vi "VI Konfiguration Kalibriergase.vi"() -> ()   [LabVIEW 2020, in "CalGas Aufschaltung.lvlib"]
uses:
  Seiten/CalGas Aufschaltung/CalGas Aufschaltung.lvlib
  Seiten/CalGas Aufschaltung/Definition CalGas Anzeige.ctl
  Seiten/CalGas Aufschaltung/CalGas-Namen.ctl
  Visualisierungs Elemente/String - Eingabefeld.ctl
  Seiten/CalGas Aufschaltung/CalGas-Werte.ctl
  Visualisierungs Elemente/Zahlen-Eingabefeld.ctl
  Seiten/CalGas Aufschaltung/CalGas-Einheit.ctl
  Visualisierungs Elemente/Auswahlfeld.ctl
  Seiten/CalGas Aufschaltung/CalGas-Messbereiche.ctl
  Seiten/CalGas Aufschaltung/Aufschaltung CalGas_ANZEIGE.ctl
  Seiten/CalGas Aufschaltung/Cluster Auswahl Analysator.ctl
  Seiten/CalGas Aufschaltung/Analysator Auswahl.ctl
  Seiten/CalGas Aufschaltung/FGV CalGas Aktionen.ctl
  Passwortverwaltung/FGV Passwort Aktion.ctl
  Analysator Definition/FGV Analysator Definition Aktionen.ctl
  Passwortverwaltung/Passwort.lvlib
  Allgemein/allgemeine Sub-VIs.lvlib
  Analysator Definition/Analysator Definition.lvlib
panel:
  in  "Analysator Auswahl":T1 {"Analysator Auswahl 12" items=["----"=100, "FT-IR"=0, "TEST"=1]; "Analysator Auswahl 11" items=["----"=100, "FT-IR"=0, "TEST"=1]; "Analysator Auswahl 10" items=["----"=100, "FT-IR"=0, "TEST"=1]; "Analysator Auswahl 9" items=["----"=100, "FT-IR"=0, "TEST"=1]; "Analysator Auswahl 8" items=["----"=100, "FT-IR"=0, "TEST"=1]; "Analysator Auswahl 7" items=["----"=100, "FT-IR"=0, "TEST"=1]; "Analysator Auswahl 6" items=["----"=100, "FT-IR"=0, "TEST"=1]; "Analysator Auswahl 5" items=["----"=100, "FT-IR"=0, "TEST"=1]; "Analysator Auswahl 4" items=["----"=100, "FT-IR"=0, "TEST"=1]; "Analysator Auswahl 3" items=["----"=100, "FT-IR"=0, "TEST"=1]; "Analysator Auswahl 2" items=["----"=100, "FT-IR"=0, "TEST"=1]; "Analysator Auswahl" items=["----"=100, "FT-IR"=0, "PMA"=1]}
  in  "Aufschaltung CalGas":T3 {"Aufschaltpunkt" items=["Filterblock", "Analyzer directly", "PNS", "Entnahme", "Gasdivider"]; "Kalibriergas" items=["Stickstoff"]}
  in  "Def.CalGas":T5 {"Messbereiche"."Messbereich 12" items=["---"]; "Messbereiche"."Messbereich 11" items=["---"]; "Messbereiche"."Messbereich 10" items=["---"]; "Messbereiche"."Messbereich 9" items=["---"]; "Messbereiche"."Messbereich 8" items=["---"]; "Messbereiche"."Messbereich 7" items=["---"]; "Messbereiche"."Messbereich 6" items=["---"]; "Messbereiche"."Messbereich 5" items=["---"]; "Messbereiche"."Messbereich 4" items=["---"]; "Messbereiche"."Messbereich 3" items=["---"]; "Messbereiche"."Messbereich 2" items=["---"]; "Messbereiche"."Messbereich 1" items=["---"]; "Einheit"."Einheit 12" items=["ppm", "%"]; "Einheit"."Einheit 11" items=["ppm", "%"]; "Einheit"."Einheit 10" items=["ppm", "%"]; "Einheit"."Einheit 9" items=["ppm", "%"]; "Einheit"."Einheit 8" items=["ppm", "%"]; "Einheit"."Einheit 7" items=["ppm", "%"]; "Einheit"."Einheit 6" items=["ppm", "%"]; "Einheit"."Einheit 5" items=["ppm", "%"]; "Einheit"."Einheit 4" items=["ppm", "%"]; "Einheit"."Einheit 3" items=["ppm", "%"]; "Einheit"."Einheit 2" items=["ppm", "%"]; "Einheit"."Einheit 1" items=["ppm", "%"]; "Werte 2"."Konzentration 12" format="%#_5g"; "Werte 2"."Konzentration 11" format="%#_5g"; "Werte 2"."Konzentration 10" format="%#_5g"; "Werte 2"."Konzentration 9" format="%#_5g"; "Werte 2"."Konzentration 8" format="%#_5g"; "Werte 2"."Konzentration 7" format="%#_5g"; "Werte 2"."Konzentration 6" format="%#_5g"; "Werte 2"."Konzentration 5" format="%#_5g"; "Werte 2"."Konzentration 4" format="%#_5g"; "Werte 2"."Konzentration 3" format="%#_5g"; "Werte 2"."Konzentration 2" format="%#_5g"; "Werte 2"."Konzentration 1" format="%#_5g"; "Werte"."Konzentration 12" format="%#_5g"; "Werte"."Konzentration 11" format="%#_5g"; "Werte"."Konzentration 10" format="%#_5g"; "Werte"."Konzentration 9" format="%#_5g"; "Werte"."Konzentration 8" format="%#_5g"; "Werte"."Konzentration 7" format="%#_5g"; "Werte"."Konzentration 6" format="%#_5g"; "Werte"."Konzentration 5" format="%#_5g"; "Werte"."Konzentration 4" format="%#_5g"; "Werte"."Konzentration 3" format="%#_5g"; "Werte"."Konzentration 2" format="%#_5g"; "Werte"."Konzentration 1" format="%#_5g"}
  # "Konfiguration Kalibriergase"
  # "Name"
  # "Einheit"
  # "Messbereich"
  # "Messbereich"
  # "Analysator"
  # "Name"
  # "Konzentration"
  # "Konzentration"
  # "Einheit"
  # "Aufschaltung Kalibriergas"
  # "Kalibriergas"
  # "Aufschaltpunkt"
  # "Analysator"
  # "Span 1"
  # "Span 2"
  # "Span 3"
  # "Span 4"
  # "Span 5"
  # "Span 6"
  # "Span 7"
  # "Span 8"
  # "Span 9"
  # "Span 10"
  # "Span 11"
  # "Span 12"
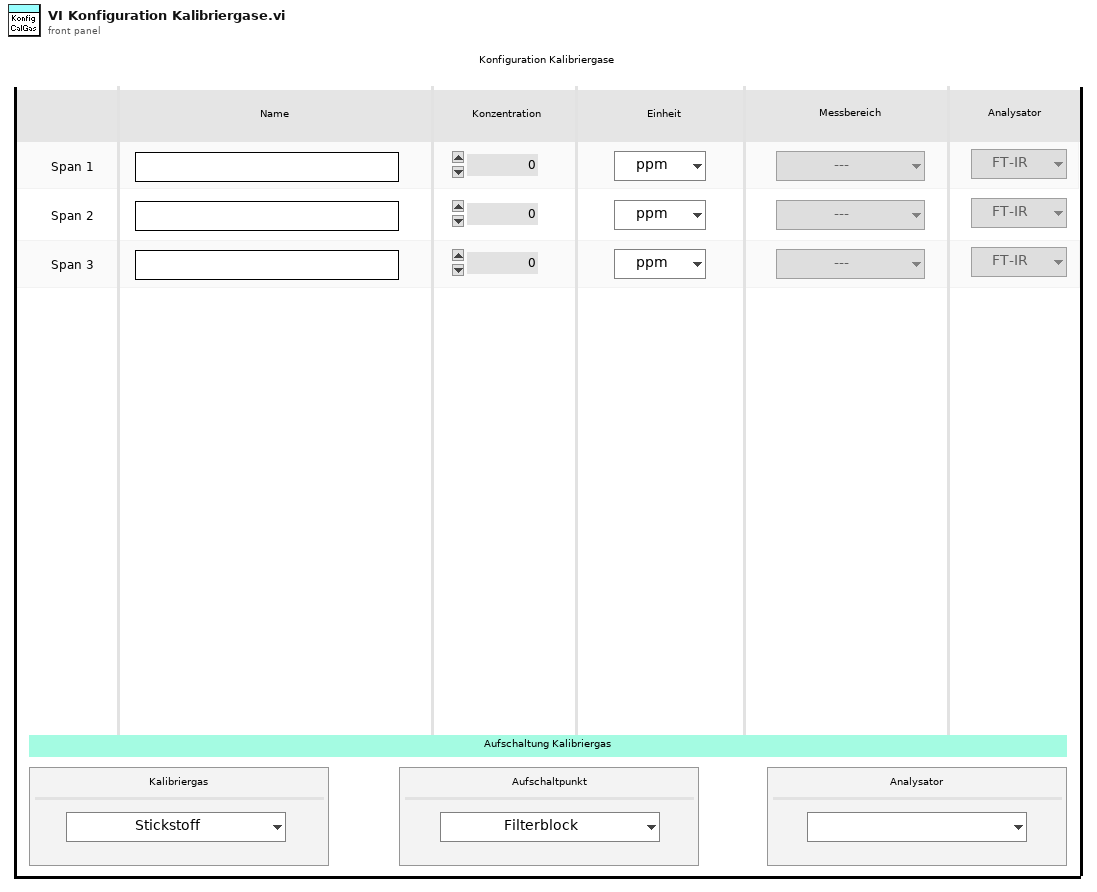
[diagram p1: front panel]
types:
  T1 = typedef "CalGas Aufschaltung.lvlib/Cluster Auswahl Analysator.ctl" = cluster{"Analysator Auswahl":T2, "Analysator Auswahl 2":T2, "Analysator Auswahl 3":T2, "Analysator Auswahl 4":T2, "Analysator Auswahl 5":T2, "Analysator Auswahl 6":T2, "Analysator Auswahl 7":T2, "Analysator Auswahl 8":T2, "Analysator Auswahl 9":T2, "Analysator Auswahl 10":T2, "Analysator Auswahl 11":T2, "Analysator Auswahl 12":T2}
  T2 = typedef "CalGas Aufschaltung.lvlib/Analysator Auswahl.ctl" = u16
  T3 = typedef "CalGas Aufschaltung.lvlib/Aufschaltung CalGas_ANZEIGE.ctl" = cluster{"Kalibriergas":T4, "Aufschaltpunkt":T4, "Analysator":T4}
  T4 = typedef "Auswahlfeld.ctl" = u16
  T5 = typedef "CalGas Aufschaltung.lvlib/Definition CalGas Anzeige.ctl" = cluster{"Namen":T6, "Werte":T8, "Werte 2":T8, "Einheit":T10, "Messbereiche":T11}
  T6 = typedef "CalGas Aufschaltung.lvlib/CalGas-Namen.ctl" = cluster{"Name":T7, "Name 2":T7, "Name 3":T7, "Name 4":T7, "Name 5":T7, "Name 6":T7, "Name 7":T7, "Name 8":T7, "Name 9":T7, "Name 10":T7, "Name 11":T7, "Name 12":T7}
  T7 = typedef "String - Eingabefeld.ctl" = string
  T8 = typedef "CalGas Aufschaltung.lvlib/CalGas-Werte.ctl" = cluster{"Konzentration 1":T9, "Konzentration 2":T9, "Konzentration 3":T9, "Konzentration 4":T9, "Konzentration 5":T9, "Konzentration 6":T9, "Konzentration 7":T9, "Konzentration 8":T9, "Konzentration 9":T9, "Konzentration 10":T9, "Konzentration 11":T9, "Konzentration 12":T9}
  T9 = typedef "Zahlen-Eingabefeld.ctl" = sgl
  T10 = typedef "CalGas Aufschaltung.lvlib/CalGas-Einheit.ctl" = cluster{"Einheit 1":T4, "Einheit 2":T4, "Einheit 3":T4, "Einheit 4":T4, "Einheit 5":T4, "Einheit 6":T4, "Einheit 7":T4, "Einheit 8":T4, "Einheit 9":T4, "Einheit 10":T4, "Einheit 11":T4, "Einheit 12":T4}
  T11 = typedef "CalGas Aufschaltung.lvlib/CalGas-Messbereiche.ctl" = cluster{"Messbereich 1":T4, "Messbereich 2":T4, "Messbereich 3":T4, "Messbereich 4":T4, "Messbereich 5":T4, "Messbereich 6":T4, "Messbereich 7":T4, "Messbereich 8":T4, "Messbereich 9":T4, "Messbereich 10":T4, "Messbereich 11":T4, "Messbereich 12":T4}
  T12 = typedef "CalGas Aufschaltung.lvlib/FGV CalGas Aktionen.ctl" = enum16{"lesen", "Analysator Auswahl", "Def.CalGas", "Aufschaltung CalGas", "laden", "speichern", "KAL extrahieren"}
  T13 = enum8{"Enabled", "Disabled", "Disabled and Grayed Out"}
  T14 = typedef "CalGas Aufschaltung.lvlib/Aufschaltung CalGas.ctl" = cluster{"Kalibriergas":T4, "Aufschaltpunkt":T15, "Analysator":T16}
  T15 = typedef "CalGas Aufschaltung.lvlib/Auswahl Aufschaltpunkt.ctl" = enum16{"über Filterblock", "Analysator direkt", "über PNS", "Entnahme", "Gasdivider"}
  T16 = typedef "CalGas Aufschaltung.lvlib/Auswahl Analysator.ctl" = enum16{"FT-IR", "FID", "PMA", "PMA/FID/FT-IR"}
  T17 = typedef "Passwort.lvlib/FGV Passwort Aktion.ctl" = enum16{"prüfen", "setzen", "Initialisieren", "PW speichern", "lesen", "PW Änderung"}
  T18 = typedef "Analysator Definition.lvlib/FGV Analysator Definition Aktionen.ctl" = enum16{"lesen", "MB setzen", "MB KAL setzen", "laden"}
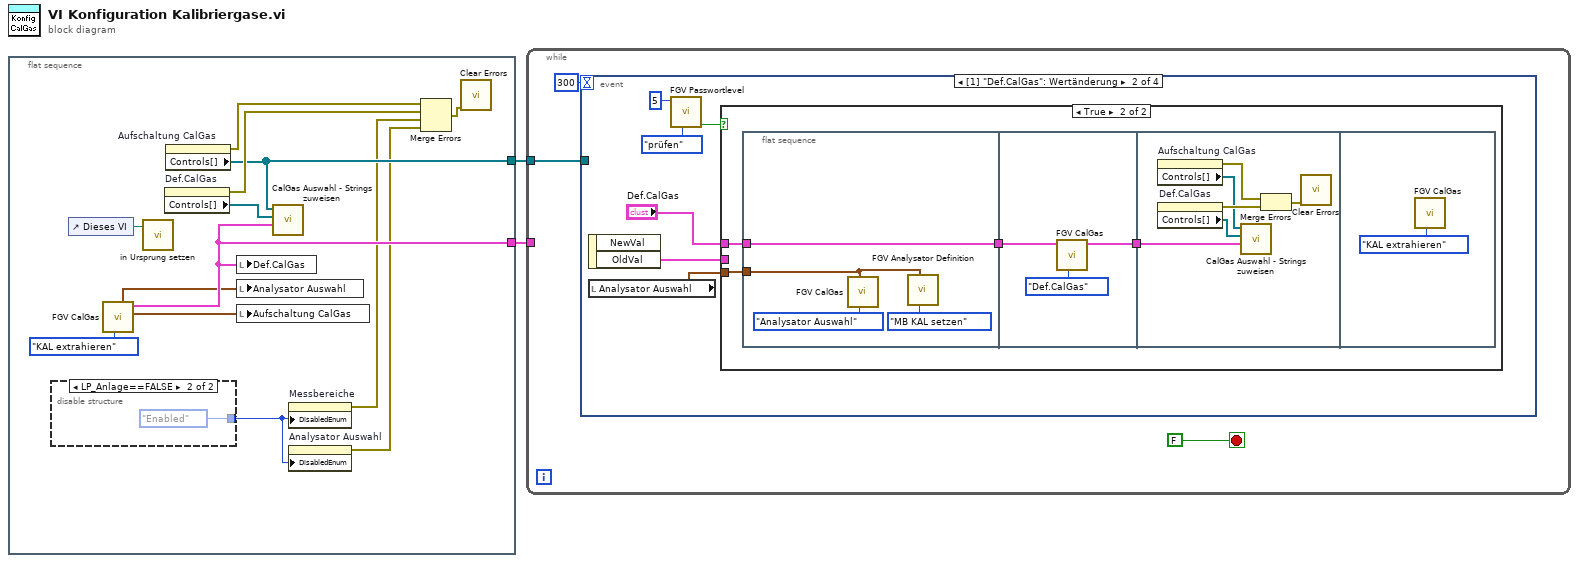
[diagram p0: block diagram]
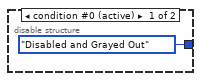
[diagram p2: hidden frame]
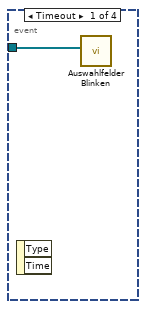
[diagram p3: hidden frame]
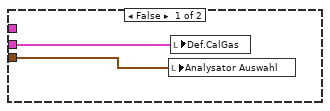
[diagram p4: hidden frame]
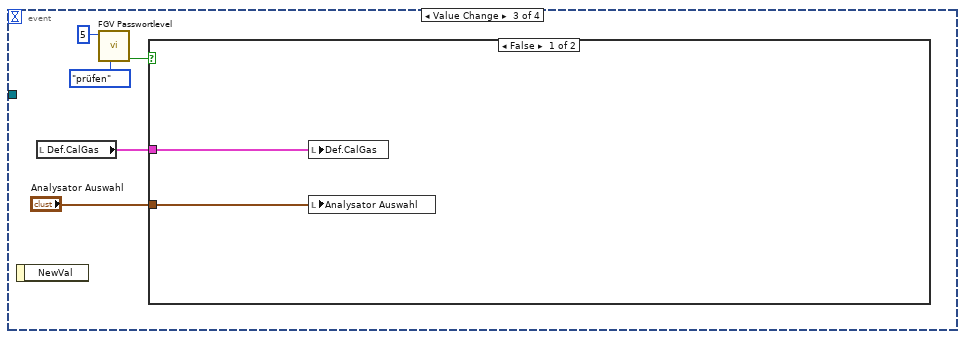
[diagram p5: hidden frame]
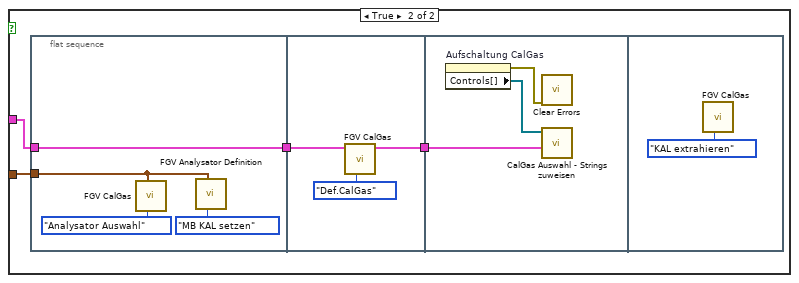
[diagram p6: hidden frame]
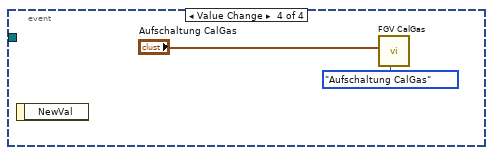
[diagram p7: hidden frame]
diagram:
  n1 = flat-sequence {
    tunnel: [w8] -> w2
    tunnel: [w13] -> w1
    frame #0 {
      n2 = disable-structure shown="LP_Anlage==FALSE" {
        disable-tunnel: [T13."Disabled and Grayed Out" ("Deaktiviert") T13."Enabled" ("Deaktiviert")] -> w3
        frame condition #0 (active) {
        }
        frame condition #1 {
        }
      }
      n3 = control-ref of="Dieses VI"() -> (w9:refnum<vi>)
      n4 = call "FGV CalGas.vi"("Aktionen"=FGV_CalGas_Aktionen."KAL extrahieren") -> ("Aufschaltung CalGas"=w7:T14, "Def.CalGas"=w8:T5, "Analysator Auswahl"=w6:T1)  [unwired: 6 in, 2 out]
      n5 = call "in Ursprung setzen.vi"("VI Referenz"=w9) -> ()  [unwired: 10 in, 1 out]
      n6 = property on="Def.CalGas" class="Cluster (strikt)"() -> (error out=w14:errorcluster, "Controls[]"=w11:refnum<vi>[])  [unwired: 2 in, 1 out]
      n7 = property on="Aufschaltung CalGas" class="Cluster (strikt)"() -> (error out=w15:errorcluster, "Controls[]"=w13:refnum<vi>[])  [unwired: 2 in, 1 out]
      n8 = local write "Def.CalGas"(w8) -> ()
      n9 = local write "Analysator Auswahl"(w6) -> ()
      n10 = local write "Aufschaltung CalGas"(w7) -> ()
      n11 = call "CalGas Auswahl - Strings zuweisen.vi"(9:"Def.CalGas"=w8, 10:"Def.CalGas"=w11, "Aufschaltung CalGas"=w13) -> ()  [unwired: 8 in, 1 out]
      n12 = property on="Messbereiche" class="Cluster (strikt)"("DisabledEnum"=w3) -> (error out=w5:errorcluster)  [unwired: 2 in, 1 out]
      n13 = property on="Analysator Auswahl" class="Cluster (strikt)"("DisabledEnum"=w3) -> (error out=w4:errorcluster)  [unwired: 2 in, 1 out]
      n14 = Merge Errors(w15, w14, w5, w4) -> (w10:errorcluster)
      n15 = call <vilib>:"Clear Errors.vi"("error in (no error)"=w10) -> ()  [unwired: 5 in, 2 out]
    }
  }
  n16 = while {
    tunnel: w2 -> [_]
    tunnel: w1 -> [w18]
    stop <- FALSE stop-if-true
    n17 = event shown="[1] \"Def.CalGas\": Wertänderung" {
      selector: _ -> [_ _ _ _]
      dyn-events: _ -> [_ _ _ _]
      timeout: 300 -> [_ _ _ _]
      tunnel: w18 -> [w21 _ _ _]
      event Timeout {
        n18 = event-data() -> ()  [unwired: 1 in, 2 out]
        n19 = call "Auswahlfelder Blinken.vi"("Controls[]"=w21) -> ()  [unwired: 11 in]
      }
      event Value Change {
        n20 = event-data() -> ("OldVal"=w22:T5)  [unwired: 1 in, 1 out]
        n21 = local read "Analysator Auswahl"() -> (w23:T1)
        n22 = call "FGV Passwortlevel.vi"("FGV Passwort Aktion"=FGV_Passwort_Aktion."prüfen", "geforderter Level"=i16 5) -> ("Freigabe"=w25:bool)  [unwired: 2 in, 7 out]
        n23 = case shown="True" w25 {
          tunnel: "Def.CalGas" -> [_ w33]
          tunnel: w23 -> [w28 w30]
          tunnel: w22 -> [w29 _]
          frame False {
            n24 = local write "Analysator Auswahl"(w28) -> ()
            n25 = local write "Def.CalGas"(w29) -> ()
          }
          frame True {
            n26 = flat-sequence {
              tunnel: w33 -> [w37]
              tunnel: [w37] -> w31
              tunnel: w30 -> [w34]
              tunnel: [w38] -> w32
              tunnel: w31 -> [w39]
              tunnel: w32 -> [w41]
              frame #0 {
                n27 = call "FGV CalGas.vi"("Aktionen"=FGV_CalGas_Aktionen."Analysator Auswahl", "Analysator Auswahl"=w34) -> ()  [unwired: 5 in, 5 out]
                n28 = call "FGV Analysator Definition.vi"("Aktionen"=FGV_Analysator_Definition_Aktionen."MB KAL setzen", "Analysator Auswahl"=w34) -> ()  [unwired: 5 in, 5 out]
              }
              frame #1 {
                n29 = call "FGV CalGas.vi"("Aktionen"=FGV_CalGas_Aktionen."Def.CalGas", "Def.CalGas neu"=w39) -> ("Def.CalGas"=w38:T5)  [unwired: 5 in, 4 out]
              }
              frame #2 {
                n30 = property on="Aufschaltung CalGas" class="Cluster (strikt)"() -> (error out=w45:errorcluster, "Controls[]"=w43:refnum<vi>[])  [unwired: 2 in, 1 out]
                n31 = property on="Def.CalGas" class="Cluster (strikt)"() -> (error out=w46:errorcluster, "Controls[]"=w44:refnum<vi>[])  [unwired: 2 in, 1 out]
                n32 = call "CalGas Auswahl - Strings zuweisen.vi"(9:"Def.CalGas"=w41, 10:"Def.CalGas"=w44, "Aufschaltung CalGas"=w43) -> ()  [unwired: 8 in, 1 out]
                n33 = Merge Errors(w45, w46) -> (w42:errorcluster)
                n34 = call <vilib>:"Clear Errors.vi"("error in (no error)"=w42) -> ()  [unwired: 5 in, 2 out]
              }
              frame #3 {
                n35 = call "FGV CalGas.vi"("Aktionen"=FGV_CalGas_Aktionen."KAL extrahieren") -> ()  [unwired: 6 in, 5 out]
              }
            }
          }
        }
      }
      event Value Change {
        n36 = event-data() -> ()  [unwired: 1 in, 1 out]
        n37 = local read "Def.CalGas"() -> (w49:T5)
        n38 = call "FGV Passwortlevel.vi"("FGV Passwort Aktion"=FGV_Passwort_Aktion."prüfen", "geforderter Level"=i16 5) -> ("Freigabe"=w50:bool)  [unwired: 2 in, 7 out]
        n39 = case shown="False" w50 {
          tunnel: w49 -> [w53 w58]
          tunnel: "Analysator Auswahl" -> [w54 w55]
          frame False {
            n40 = local write "Def.CalGas"(w53) -> ()
            n41 = local write "Analysator Auswahl"(w54) -> ()
          }
          frame True {
            n42 = flat-sequence {
              tunnel: w58 -> [w62]
              tunnel: [w62] -> w56
              tunnel: w55 -> [w59]
              tunnel: [w63] -> w57
              tunnel: w56 -> [w64]
              tunnel: w57 -> [w66]
              frame #0 {
                n43 = call "FGV CalGas.vi"("Aktionen"=FGV_CalGas_Aktionen."Analysator Auswahl", "Analysator Auswahl"=w59) -> ()  [unwired: 5 in, 5 out]
                n44 = call "FGV Analysator Definition.vi"("Aktionen"=FGV_Analysator_Definition_Aktionen."MB KAL setzen", "Analysator Auswahl"=w59) -> ()  [unwired: 5 in, 5 out]
              }
              frame #1 {
                n45 = call "FGV CalGas.vi"("Aktionen"=FGV_CalGas_Aktionen."Def.CalGas", "Def.CalGas neu"=w64) -> ("Def.CalGas"=w63:T5)  [unwired: 5 in, 4 out]
              }
              frame #2 {
                n46 = property on="Aufschaltung CalGas" class="Cluster (strikt)"() -> (error out=w68:errorcluster, "Controls[]"=w67:refnum<vi>[])  [unwired: 2 in, 1 out]
                n47 = call <vilib>:"Clear Errors.vi"("error in (no error)"=w68) -> ()  [unwired: 5 in, 2 out]
                n48 = call "CalGas Auswahl - Strings zuweisen.vi"("Def.CalGas"=w66, "Aufschaltung CalGas"=w67) -> ()  [unwired: 9 in, 1 out]
              }
              frame #3 {
                n49 = call "FGV CalGas.vi"("Aktionen"=FGV_CalGas_Aktionen."KAL extrahieren") -> ()  [unwired: 6 in, 5 out]
              }
            }
          }
        }
      }
      event Value Change {
        n50 = event-data() -> ()  [unwired: 1 in, 1 out]
        n51 = call "FGV CalGas.vi"("Aktionen"=FGV_CalGas_Aktionen."Aufschaltung CalGas", "Aufschaltung CalGas"="Aufschaltung CalGas") -> ()  [unwired: 5 in, 5 out]
      }
    }
  }
